vi "Read Count Measurement (Serial Bus - A429).vi"(8 "error in (no error)":errorcluster, 10 "Serial Bus Name (1: Serial Bus 1)":i32(ring)=1 items=["Serial Bus 1"=1, "Serial Bus 2"=2], 11 "VISA resource name":refnum<visa-resource-name>) -> (0 "error out":errorcluster, 1 "Word Count":dbl, 2 "Error Count":dbl, 3 "VISA resource name out":refnum<visa-resource-name>)   [LabVIEW 2017, in "Agilent 2000 3000 X-Series.lvlib"]
doc: "Returns the measurement of serial bus - ARINC 429.\n\nNote:\nThis VI is not supported by EDUX1052A/G, DSOX1202A/G, DSOX1204A/G models"
uses:
  Agilent 2000 3000 X-Series.lvlib
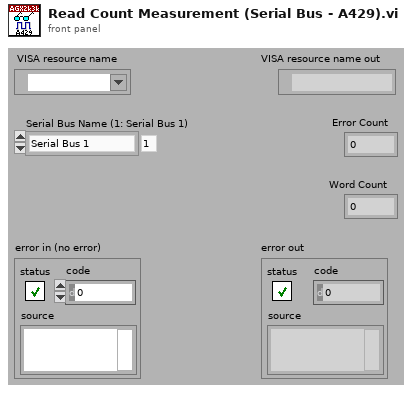
[diagram p1: front panel]
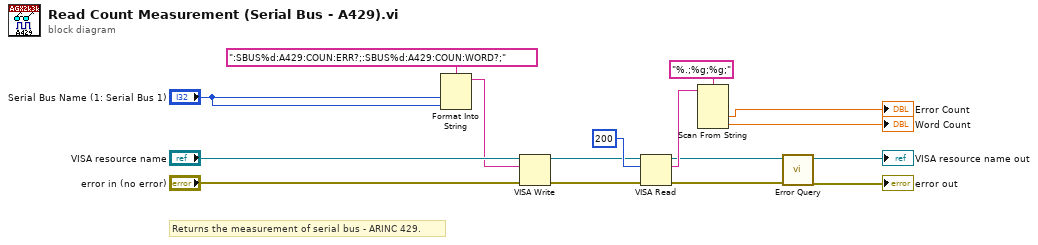
[diagram p0: block diagram]
diagram:
  # "Returns the measurement of serial bus - ARINC 429."
  n1 = Format Into String(format string=":SBUS%d:A429:COUN:ERR?;:SBUS%d:A429:COUN:WORD?;", "Serial Bus Name (1: Serial Bus 1)", "Serial Bus Name (1: Serial Bus 1)") -> (resulting string=w4:string)  [unwired: 2 in, 1 out]
  n2 = VISA Write(VISA resource name="VISA resource name", write buffer=w4, error in (no error)="error in (no error)") -> (VISA resource name out=w8:refnum<visa-resource-name>, error out=w7:errorcluster)  [unwired: 1 out]
  n3 = VISA Read(VISA resource name=w8, byte count=u32 200, error in (no error)=w7) -> (VISA resource name out=w5:refnum<visa-resource-name>, read buffer=w10:string, error out=w6:errorcluster)  [unwired: 1 out]
  n4 = Scan From String(format string="%.;%g;%g;", input string=w10) -> (output 1=→"Error Count":dbl, output 2=→"Word Count":dbl)  [unwired: 2 in, 5 out]
  n5 = call "Error Query.vi"("error in (no error)"=w6, "VISA resource name"=w5) -> ("error out"=→"error out":errorcluster, "VISA resource name out"=→"VISA resource name out":refnum<visa-resource-name>)  [unwired: 8 out]
